vi "testBuildStateStringwithArgumentsExecutionPriority.vi"(8 "error in (no error)":errorcluster, 11 "testStateMachineUtilities in":refnum<class "testStateMachineUtilities.lvclass">) -> (0 "error out":errorcluster, 3 "testStateMachineUtilities out":refnum<class "testStateMachineUtilities.lvclass">)   [LabVIEW 2020, in "testStateMachineUtilities.lvclass"]
uses:
  testStateMachineUtilities.lvclass
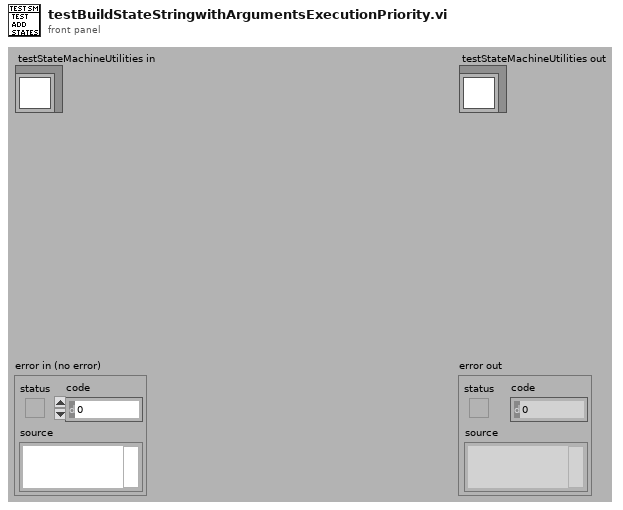
[diagram p1: front panel]
types:
  T1 = enum32{"invalid priority", "background priority", "normal priority", "above normal priority", "high priority", "time critical priority", "subroutine"}
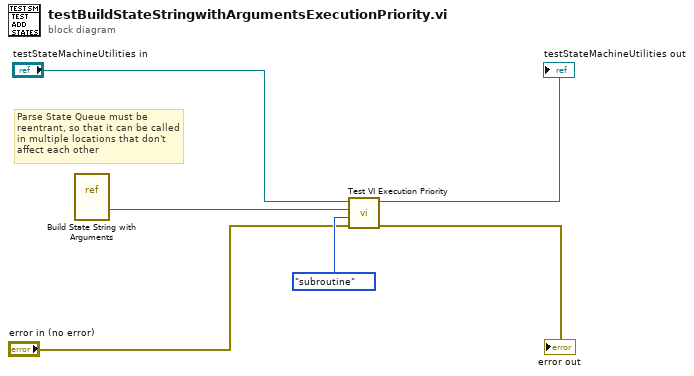
[diagram p0: block diagram]
diagram:
  # "Parse State Queue must be reentrant, so that it can be called in multiple locations that don't affect each other"
  n1 = vi-ref "Build State String with Arguments.vi"() -> (w1:refnum<vi>)
  n2 = call "Test VI Execution Priority.vi"("error in (no error)"="error in (no error)", "Execution:Priority"=T1."subroutine", "VI Refnum"=w1, "testStateMachineUtilities in"="testStateMachineUtilities in") -> ("error out"=→"error out":errorcluster, "testStateMachineUtilities out"=→"testStateMachineUtilities out":refnum<class "testStateMachineUtilities.lvclass">)  [unwired: 6 in]
